vi "State Entry.vi"(8 "error in (no error)":errorcluster, 11 "View Model":T1) -> (0 "error out":errorcluster, 3 "View Model":T1)   [LabVIEW 2017]
doc: "Process transition between elevator sonctroller states."
uses:
  View Model/Controls/View Model.ctl
  View Model/Controls/Shared Model.ctl
  Error Handler/Controls/Error Model.ctl
  Error Handler/Controls/Error Data.ctl
  Error Handler/Controls/Error Level.ctl
  Configuration/Controls/Config Model.ctl
  Configuration/Controls/Config Data Record.ctl
  Configuration/Controls/Config Command.ctl
  Controls/Control Model.ctl
  Controls/Elevator Location.ctl
  Controls/Elevator Status.ctl
  Controls/Control Event.ctl
  Controls/Control CMD.ctl
  Controls/Controller - Overhead.ctl
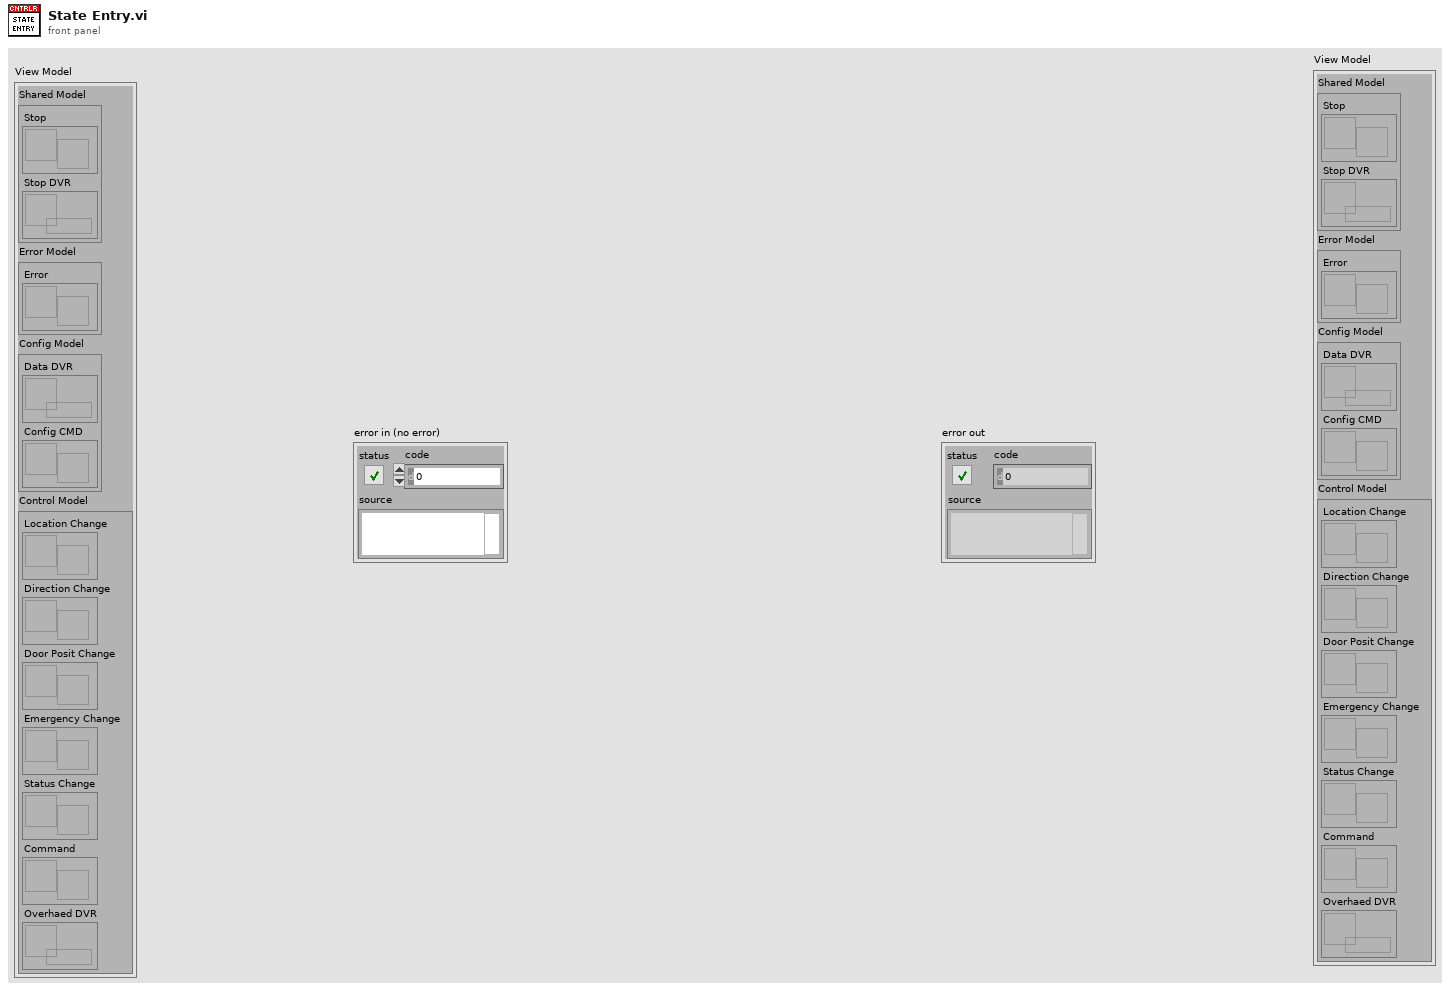
[diagram p1: front panel]
types:
  T1 = typedef "View Model.ctl" = cluster{"Shared Model":T2, "Error Model":T3, "Config Model":T4, "Control Model":T5}
  T2 = typedef "Shared Model.ctl" = cluster{"Stop":refnum<user-event>, "Stop DVR":refnum<data-value>}
  T3 = typedef "Error Model.ctl" = cluster{"Error":refnum<user-event>}
  T4 = typedef "Config Model.ctl" = cluster{"Data DVR":refnum<data-value>, "Config CMD":refnum<user-event>}
  T5 = typedef "Control Model.ctl" = cluster{"Location Change":refnum<user-event>, "Direction Change":refnum<user-event>, "Door Posit Change":refnum<user-event>, "Emergency Change":refnum<user-event>, "Status Change":refnum<user-event>, "Command":refnum<user-event>, "Overhaed DVR":refnum<data-value>}
  T6 = typedef "Elevator Status.ctl" = enum16{"No Request", "Initial", "Wait for 1st Request", "Start and Move", "Continue Move", "Analysis", "Stop at Floor", "Open/Close Door", "Emergency Call", "Terminate"}
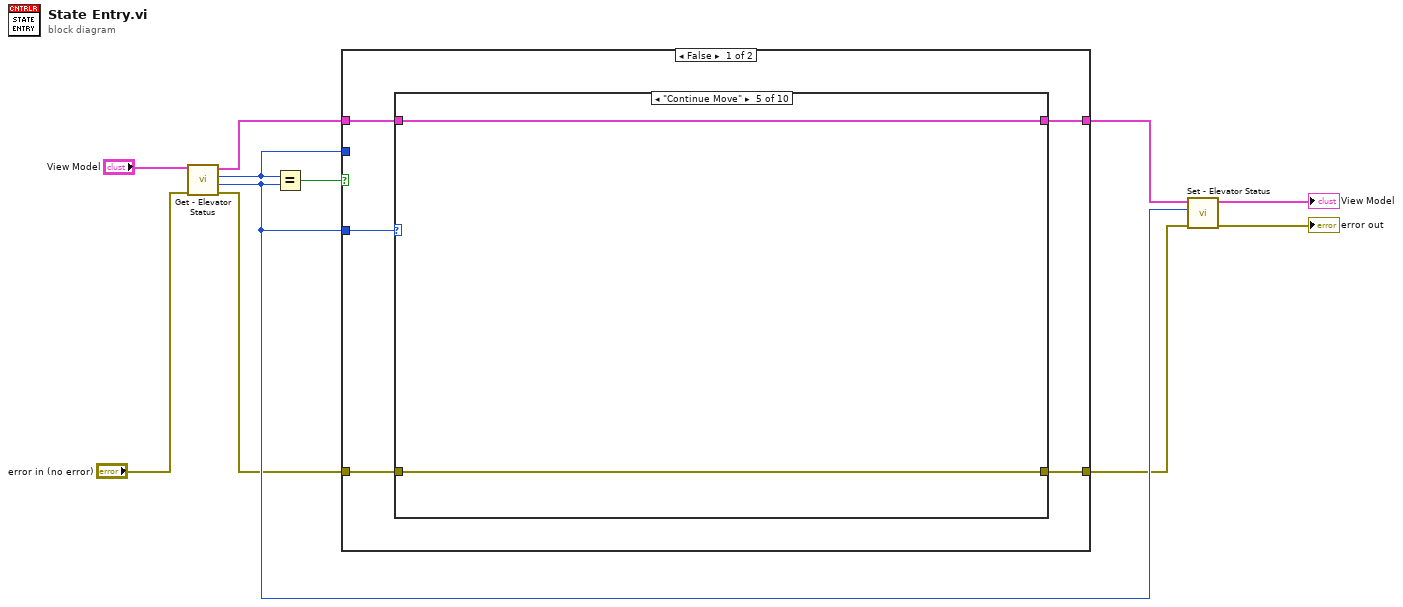
[diagram p0: block diagram]
diagram:
  n1 = call "Get - Elevator Status.vi"("error in (no error)"="error in (no error)", "View Model"="View Model") -> ("error out"=w1:errorcluster, "Next Status"=w8:T6, "Current Status"=w9:T6, "View Model"=w7:T1)  [unwired: 6 in]
  n2 = Equal?(x=w9, y=w8) -> (x = y?=w10:bool)
  n3 = case shown="False" w10 {
    tunnel: w9 -> [_ _]
    tunnel: w8 -> [w16 _]
    tunnel: w7 -> [w15 w38]
    tunnel: [w14 w38] -> w6
    tunnel: w1 -> [w13 w37]
    tunnel: [w12 w37] -> w2
    frame False {
      n4 = case shown="\"Continue Move\"" w16 {
        tunnel: w15 -> [w18 w20 w22 w24 w26 w28 w30 w32 w34 w36]
        tunnel: [w18 w20 w22 w24 w26 w28 w30 w32 w34 w36] -> w14
        tunnel: w13 -> [w17 w19 w21 w23 w25 w27 w29 w31 w33 w35]
        tunnel: [w17 w19 w21 w23 w25 w27 w29 w31 w33 w35] -> w12
        frame "No Request", Default {
        }
        frame "Initial" {
        }
        frame "Wait for 1st Request" {
        }
        frame "Start and Move" {
          # "[Covers: SS1]"
          # "#TODO\nTransition to next state - Open/Close Door"
        }
        frame "Continue Move" {
        }
        frame "Analysis" {
          # "[Covers: AS1]"
          # "#TODO\nRead values of all User Controls GUI controls\nand Elevator Location from DVR.\nRealize undefined Get DVR values based on Template DVR"
        }
        frame "Stop at Floor" {
        }
        frame "Open/Close Door" {
        }
        frame "Emergency Call" {
        }
        frame "Terminate" {
        }
      }
    }
    frame True {
    }
  }
  n5 = call "Set - Elevator Status.vi"("error in (no error)"=w2, "Current Status"=w8, "View Model"=w6) -> ("error out"=→"error out":errorcluster, "View Model"=→"View Model":T1)  [unwired: 7 in]
